vi "Shift.vi"() -> (7 "Shift":string)   [LabVIEW 2017]
panel:
  out "time string":string
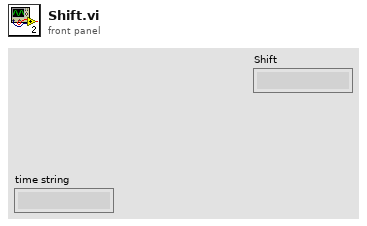
[diagram p1: front panel]
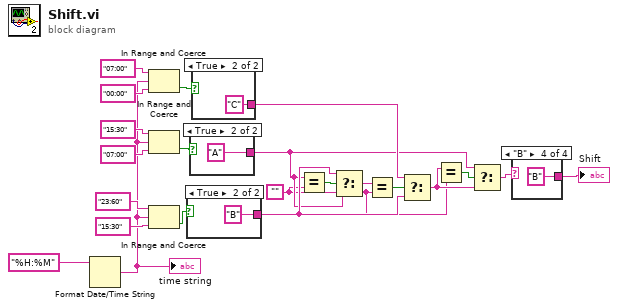
[diagram p0: block diagram]
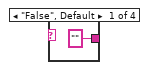
[diagram p2: hidden frame]
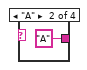
[diagram p3: hidden frame]
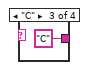
[diagram p4: hidden frame]
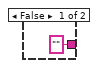
[diagram p5: hidden frame]
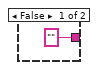
[diagram p6: hidden frame]
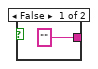
[diagram p7: hidden frame]
diagram:
  w4 = ""
  n1 = Format Date/Time String(time format string (%c)="%H:%M") -> (date/time string=w1:string)  [unwired: 2 in]
  "time string" <- w1
  n2 = In Range and Coerce(upper limit="07:00" ("String"), x=w1, lower limit="00:00" ("String")) -> (In Range?=w14:bool)  [unwired: 1 out]
  n3 = In Range and Coerce(upper limit="15:30" ("String"), x=w1, lower limit="07:00" ("String")) -> (In Range?=w20:bool)  [unwired: 1 out]
  n4 = In Range and Coerce(upper limit="23:60" ("String"), x=w1, lower limit="15:30" ("String")) -> (In Range?=w17:bool)  [unwired: 1 out]
  n5 = case shown="True" w17 {
    tunnel: ["" ("String") "B" ("String")] -> w9
    frame False {
    }
    frame True {
    }
  }
  n6 = case shown="True" w20 {
    tunnel: ["" ("String") "A" ("String")] -> w7
    frame False {
    }
    frame True {
    }
  }
  n7 = case shown="True" w14 {
    tunnel: ["" ("String") "C" ("String")] -> w10
    frame False {
    }
    frame True {
    }
  }
  n8 = Equal?(x=w7, y=w4) -> (x = y?=w13:bool)
  n9 = Select(t=w9, s=w13, f=w7) -> (s? t:f=w12:string)
  n10 = Equal?(x=w12, y=w4) -> (x = y?=w11:bool)
  n11 = Select(t=w10, s=w11, f=w9) -> (s? t:f=w6:string)
  n12 = Equal?(x=w6, y=w4) -> (x = y?=w8:bool)
  n13 = Select(t=w7, s=w8, f=w6) -> (s? t:f=w5:string)
  n14 = case shown="\"B\"" w5 {
    tunnel: ["" ("String") "A" ("String") "C" ("String") "B" ("String")] -> w3
    frame "False", Default {
    }
    frame "A" {
    }
    frame "C" {
    }
    frame "B" {
    }
  }
  "Shift" <- w3
